vi "Finalize.vi"(8 "error in":errorcluster, 11 "Tx UDP Execution Unit in":refnum<class "Tx UDP Execution Unit.lvclass">) -> (0 "error out":errorcluster, 3 "Tx UDP Execution Unit out":refnum<class "Tx UDP Execution Unit.lvclass">)   [LabVIEW 2020, in "AIM ARINC 664 Engine.lvlib" / "Implementation.lvlib" / "Tx UDP Execution Unit.lvclass"]
uses:
  Tx UDP Execution Unit.lvclass
  Tx UDP Execution Unit.lvclass/Tx UDP Execution Unit.ctl
  <instrlib>/AIM GmbH/_AIM 664/bsp/Fdx Stop (Tx).vi
  <instrlib>/AIM GmbH/_AIM 664/AIM664LV.lvlib
  <vilib>/Utility/SystemLogging/NI_SystemLogging.lvlib
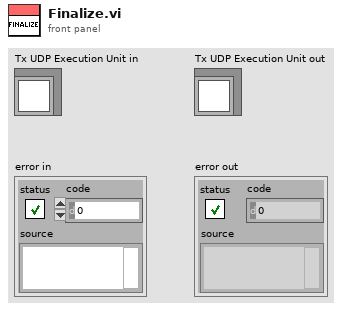
[diagram p1: front panel]
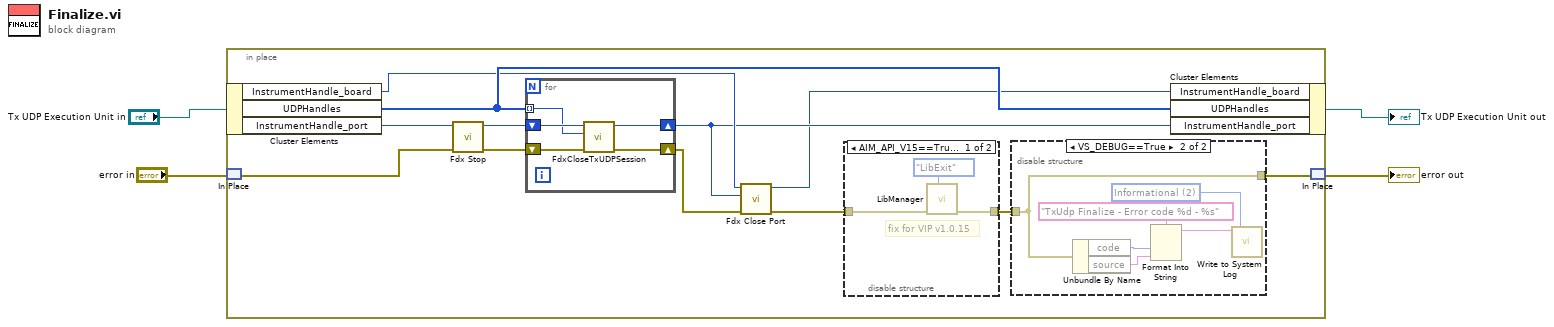
[diagram p0: block diagram]
diagram:
  n1 = in-place {
    n2 = in-place-cluster #1("Tx UDP Execution Unit in") -> ("InstrumentHandle_board"=w10:u32, "UDPHandles"=w12:u32[], "InstrumentHandle_port"=w13:u32)
    n3 = in-place-match #2("error in") -> (w14:errorcluster)
    n4 = call-poly <instrlib>:"Fdx Stop.vi"("error in"=w14, "InstrumentHandle_port in"=w13) -> ("error out"=w15:errorcluster, "InstrumentHandle_port out"=w16:u32)  [unwired: 8 in]
    n5 = for {
      shift-right: [w29] -> w9
      shift-left: w16 -> [w32]
      shift-right: [w30] -> w11
      shift-left: w15 -> [w31]
      tunnel: w12 -> [w28] mode=indexing
      n6 = call <instrlib>:"FdxCloseTxUDPSession.vi"("error in"=w31, "UdpHandle"=w28, "InstrumentHandle"=w32) -> ("error out"=w30:errorcluster, "InstrumentHandle"=w29:u32)  [unwired: 7 in]
    }
    n7 = call <instrlib>:"Fdx Close Port.vi"("error in"=w11, "InstrumentHandle_port in"=w9, "InstrumentHandle_board in"=w10) -> ("error out"=w8:errorcluster, "InstrumentHandle_board out"=w7:u32)  [unwired: 7 in]
    n8 = disable-structure shown="AIM_API_V15==True" {
      disable-tunnel: w8 -> [w19 w20]
      disable-tunnel: [w18 w20] -> w6
      frame condition #0 {
        # "fix for VIP v1.0.15"
        n9 = call <instrlib>:"LibManager.vi"("action"=enum16{"LibInit", "LibExit"}."LibExit", "error in (no error)"=w19) -> ("error out"=w18:errorcluster)  [unwired: 7 in, 2 out]
      }
      frame condition #1 (active) {
      }
    }
    n10 = disable-structure shown="VS_DEBUG==True" {
      disable-tunnel: w6 -> [w21 w22]
      disable-tunnel: [w21 w22] -> w5
      frame condition #0 (active) {
      }
      frame condition #1 {
        w25 = 2 items=["Error", "Warning", "Informational"] ("severity")
        n11 = Unbundle By Name(w22) -> ("code"=w24:i32, "source"=w23:string)
        n12 = Format Into String(format string="TxUdp Finalize - Error code %d - %s", w24, w23) -> (resulting string=w26:string)  [unwired: 2 in, 1 out]
        n13 = call <vilib>:"Write to System Log.vi"("severity"=w25, "message"=w26) -> ()  [unwired: 9 in, 1 out]
      }
    }
    n14 = in-place-cluster #1("InstrumentHandle_board"=w7, "UDPHandles"=w12, "InstrumentHandle_port"=w9) -> (→"Tx UDP Execution Unit out":refnum<class "Tx UDP Execution Unit.lvclass">)
    n15 = in-place-match #2(w5) -> (→"error out":errorcluster)
  }
